vi "AvailableElements.vi"(1 "Array":i32[](array[numeric])) -> (4 "No Available":i32, 5 "Occupied":i32[](array[numeric]))   [LabVIEW 2013]
doc: "This vi returns the number of zero elements in the input vector"
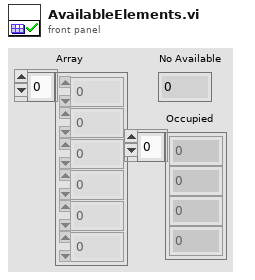
[diagram p1: front panel]
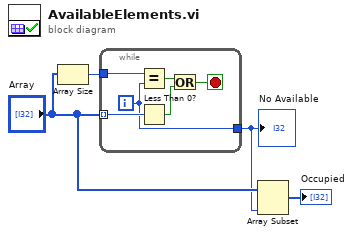
[diagram p0: block diagram]
diagram:
  n1 = Array Size(array="Array") -> (size(s)=w4:i32)
  n2 = while {
    tunnel: [w7] -> w1
    tunnel: "Array" -> [w10] mode=indexing
    tunnel: w4 -> [w8]
    i -> [w7]
    stop <- w6 stop-if-true
    n3 = Equal?(x=w8, y=w7) -> (x = y?=w5:bool)
    n4 = Less Than 0?(x=w10) -> (x < 0?=w9:bool)
    n5 = Or(x=w5, y=w9) -> (x .or. y?=w6:bool)
  }
  "No Available" <- w1
  n6 = Array Subset(array="Array", length=w1) -> (→"Occupied":i32[])  [unwired: 1 in]
